vi "KE622x -- 2182 -A Get Digital Filter Type.vi"(0 "622x Resource In":refnum<visa-resource-name>, 1 "Check For SCPI Errors? (T)":bool=TRUE, 11 "error in (no error)":errorcluster) -> (4 "622x Resource Out (dupl)":refnum<visa-resource-name>, 8 "Filter Type":T1=enum."Repeat", 15 "error out":errorcluster)   [LabVIEW 2019, in "Keithley 622x.lvlib"]
uses:
  Keithley 622x.lvlib
  Typedefs/KE2182 -- Filter Type.ctl
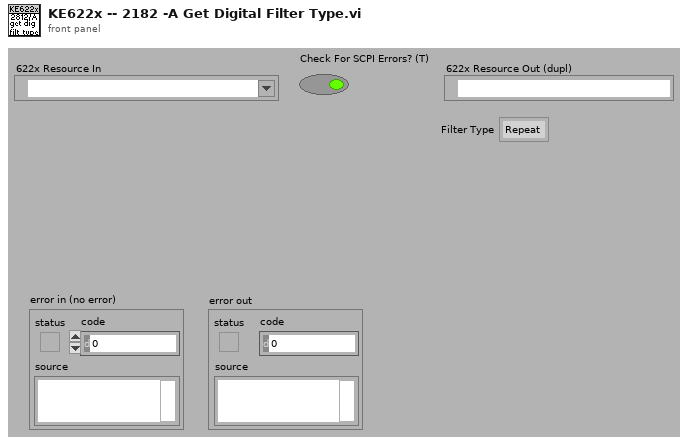
[diagram p1: front panel]
types:
  T1 = typedef "Keithley 622x.lvlib/KE2182 -- Filter Type.ctl" = enum16{"Moving", "Repeat"}
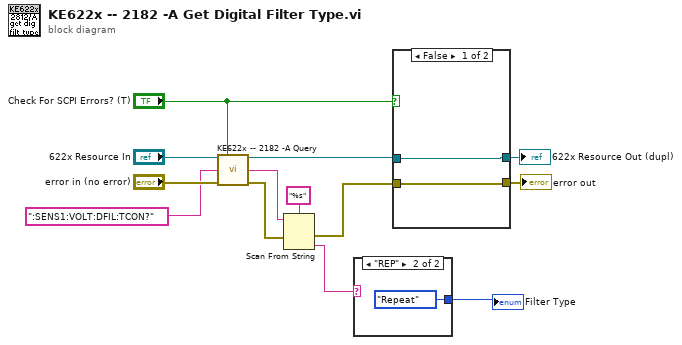
[diagram p0: block diagram]
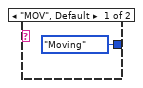
[diagram p2: hidden frame]
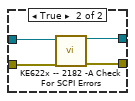
[diagram p3: hidden frame]
diagram:
  n1 = call "KE622x -- 2182 -A Query.vi"("622x Resource In"="622x Resource In", "Check For SCPI Errors? (T)"="Check For SCPI Errors? (T)", "2182-A Write String"=":SENS1:VOLT:DFIL:TCON?", "error in (no error)"="error in (no error)") -> ("622x Resource Out (dupl)"=w7:refnum<visa-resource-name>, "2182-A Reponse String"=w8:string, "error out"=w10:errorcluster)  [unwired: 9 in]
  n2 = Scan From String(format string="%s", input string=w8, error in=w10) -> (error out=w6:errorcluster, output 1=w2:string)  [unwired: 2 in, 2 out]
  n3 = case shown="\"REP\"" w2 {
    tunnel: [KE2182_--_Filter_Type."Moving" ("Filter Type") KE2182_--_Filter_Type."Repeat" ("Filter Type")] -> w1
    frame "MOV", Default {
    }
    frame "REP" {
    }
  }
  "Filter Type" <- w1
  n4 = case shown="False" "Check For SCPI Errors? (T)" {
    tunnel: w7 -> [w17 w21]
    tunnel: w6 -> [w16 w20]
    tunnel: [w17 w19] -> w4
    tunnel: [w16 w18] -> w3
    frame False {
    }
    frame True {
      n5 = call "KE622x -- 2182 -A Check For SCPI Errors.vi"("VISA Resource In"=w21, "error in (no error)"=w20) -> ("VISA Resource Out (dupl)"=w19:refnum<visa-resource-name>, "error out"=w18:errorcluster)  [unwired: 10 in, 2 out]
    }
  }
  "622x Resource Out (dupl)" <- w4
  "error out" <- w3
